vi "SNMP Build Get Request Packet.vi"(2 "Community Name":string="public", 3 "OID ARRAY":string[](array[string])) -> (0 "SNMP Packet":u8[](array[numeric]) format="%.0x", 1 "RequestID":u16 format="%.0x")   [LabVIEW 2017]
doc: "This VI constructs an SNMP Get Request. It requires an OID array and a Community Name as input. The VI returns the Request ID of the packet and the SNMP packet itself (as a byte array)."
uses:
  CTL - SNMP Types.ctl
panel:
  in  "SNMP Data Types":T1={"Integer"=2, "Octet-String"=4, "NULL"=5, "Object Identifier"=6, "Sequence"=48, "IP Address"=64, "Counter"=65, "Gauge"=66, "TimeTicks"=67, "Opaque"=68, "GetRequest-PDU"=160, "GetNextRequest-PDU"=161, "GetResponse-PDU"=162, "SetRequest-PDU"=163, "Trap-PDU"=164} {"Opaque" format="%.0x"; "TimeTicks" format="%.0x"; "Gauge" format="%.0x"; "Counter" format="%.0x"; "IP Address" format="%.0x"; "NULL" format="%.0x"; "Trap-PDU" format="%.0x"; "SetRequest-PDU" format="%.0x"; "GetNextRequest-PDU" format="%.0x"; "Object Identifier" format="%.0x"; "Sequence" format="%.0x"; "GetResponse-PDU" format="%.0x"; "GetRequest-PDU" format="%.0x"; "Octet-String" format="%.0x"; "Integer" format="%.0x"}
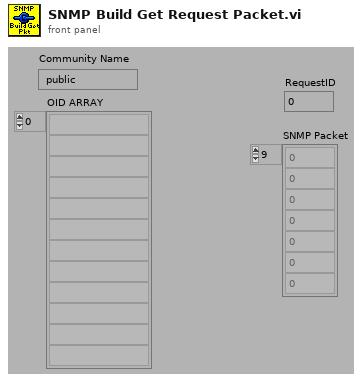
[diagram p1: front panel]
types:
  T1 = typedef "CTL - SNMP Types.ctl" = cluster{"Integer":u8, "Octet-String":u8, "NULL":u8, "Object Identifier":u8, "Sequence":u8, "IP Address":u8, "Counter":u8, "Gauge":u8, "TimeTicks":u8, "Opaque":u8, "GetRequest-PDU":u8, "GetNextRequest-PDU":u8, "GetResponse-PDU":u8, "SetRequest-PDU":u8, "Trap-PDU":u8}
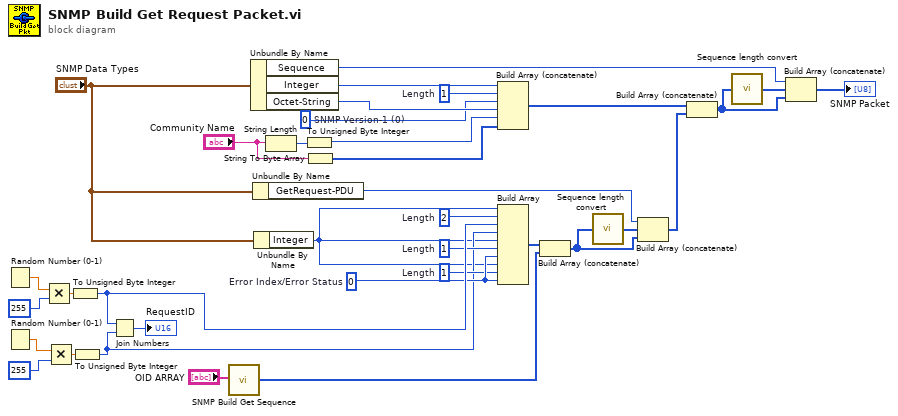
[diagram p0: block diagram]
diagram:
  w33 = u8 0  # Error Index/Error Status
  w20 = u8 0  # SNMP Version-1 (0)
  w28 = u8 1  # Length
  w29 = u8 1  # Length
  w30 = u8 2  # Length
  w32 = u8 1  # Length
  n1 = Random Number (0-1)() -> (number: 0 to 1=w18:dbl)
  n2 = Random Number (0-1)() -> (number: 0 to 1=w15:dbl)
  n3 = Multiply(x=w18, y=255) -> (x*y=w26:dbl)
  n4 = Multiply(x=w15, y=255) -> (x*y=w17:dbl)
  n5 = To Unsigned Byte Integer(number=w26) -> (unsigned 8bit integer=w34:u8)
  n6 = To Unsigned Byte Integer(number=w17) -> (unsigned 8bit integer=w14:u8)
  n7 = Join Numbers(hi=w34, lo=w14) -> ((hi.lo)=→"RequestID":u16)
  n8 = call "SNMP Build Get Sequence.vi"("OID ARRAY"="OID ARRAY") -> ("SequenceArray"=w2:u8[])
  n9 = Unbundle By Name("SNMP Data Types") -> ("Sequence"=w19:u8, "Integer"=w10:u8, "Octet-String"=w31:u8)
  n10 = Unbundle By Name("SNMP Data Types") -> ("GetRequest-PDU"=w9:u8)
  n11 = Unbundle By Name("SNMP Data Types") -> ("Integer"=w4:u8)
  n12 = String Length(string="Community Name") -> (length=w25:i32)
  n13 = To Unsigned Byte Integer(number=w25) -> (unsigned 8bit integer=w12:u8)
  n14 = String To Byte Array(string="Community Name") -> (unsigned byte array=w11:u8[])
  n15 = Build Array (concatenate)(w10, w32, w20, w31, w12, w11) -> (w22:u8[])
  n16 = Build Array(w4, w30, w34, w14, w4, w29, w33, w4, w28, w33) -> (w24:u8[])
  n17 = Build Array (concatenate)(w24, w2) -> (w8:u8[])
  n18 = call "Sequence length convert.vi"("Sequence"=w8) -> ("Sequence Length"=w23:u8[])  [unwired: 4 out]
  n19 = Build Array (concatenate)(w9, w23, w8) -> (w7:u8[])
  n20 = Build Array (concatenate)(w22, w7) -> (w6:u8[])
  n21 = call "Sequence length convert.vi"("Sequence"=w6) -> ("Sequence Length"=w21:u8[])  [unwired: 4 out]
  n22 = Build Array (concatenate)(w19, w21, w6) -> (→"SNMP Packet":u8[])
